vi "hydraharp_write_record_type.vi"(8 "error in (no error)":errorcluster, 10 "Record Type":T1, 11 "hydraharp in":refnum<class "hydraharp.lvclass">) -> (0 "error out":errorcluster, 3 "hydraharp out":refnum<class "hydraharp.lvclass">)   [LabVIEW 2015, in "hydraharp.lvclass"]
uses:
  hydraharp.lvclass
  record_type.ctl
  hydraharp.lvclass/hydraharp.ctl
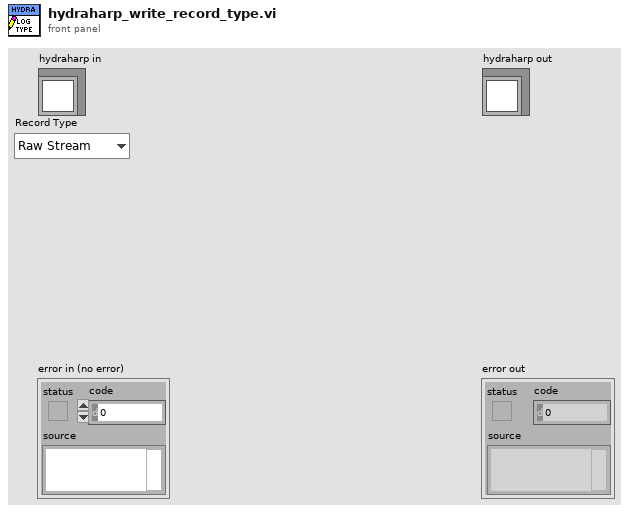
[diagram p1: front panel]
types:
  T1 = typedef "record_type.ctl" = enum16{"Raw Stream", "Processed Records (hdf5)"}
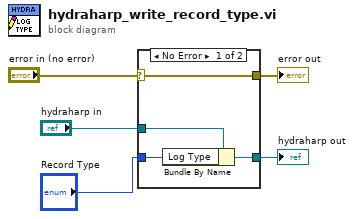
[diagram p0: block diagram]
diagram:
  n1 = case shown="No Error" "error in (no error)" {
    selector: "error in (no error)" -> [w9 w10]
    tunnel: [w9 w10] -> w4
    tunnel: [w7 w11] -> w2
    tunnel: "hydraharp in" -> [w8 w11]
    tunnel: "Record Type" -> [w6 _]
    frame No Error {
      n2 = Bundle By Name(cluster=w8, "Log Type"=w6) -> (w7:refnum<class "hydraharp.lvclass">)
    }
    frame Error {
    }
  }
  "error out" <- w4
  "hydraharp out" <- w2
